vi "Send and Receive Example.vi"(0 "Input Data":T1 {"Command" format="%02x"; "Destination" format="%02x"; "Source" format="%02x"}, 1 "Read Timeout (ms)":u32=500, 5 "Expected Command":string=".*", 7 "Expected Data":string=".*", 11 "Error In":errorcluster) -> (4 "Raw Data Out":string, 6 "Coverted Data Out":T2 {"CRC" format="%04x"; "Length" format="%02x"; "Command" format="%02x"; "Destination" format="%02x"; "Source" format="%02x"}, 15 "Error Out":errorcluster)   [LabVIEW 2016]
doc: "This standalone VI sends a GEA2 message and returns the very next response."
uses:
  type defs/Data Out.ctl
  type defs/Data In.ctl
  library/GEA2_Toolkit.lvlib
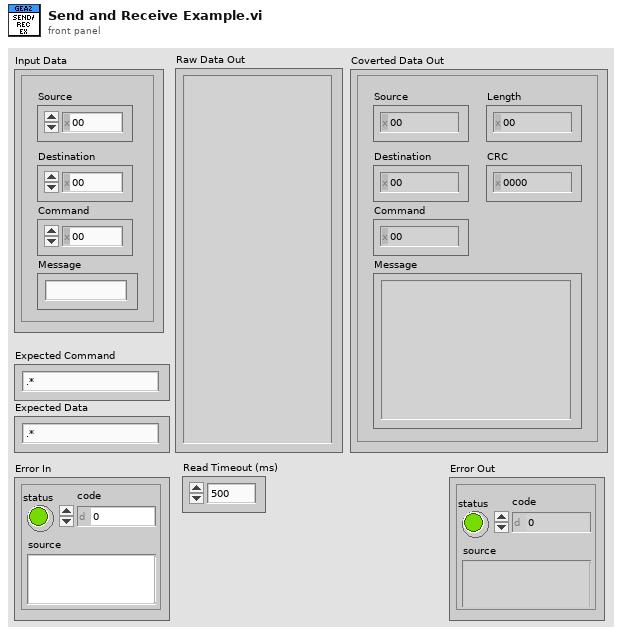
[diagram p1: front panel]
types:
  T1 = typedef "GEA2_Toolkit.lvlib/Data In.ctl" = cluster{"Source":u8, "Destination":u8, "Command":u8, "Message":string}
  T2 = typedef "GEA2_Toolkit.lvlib/Data Out.ctl" = cluster{"Source":u8, "Destination":u8, "Command":u8, "Length":u8, "CRC":u16, "Message":string}
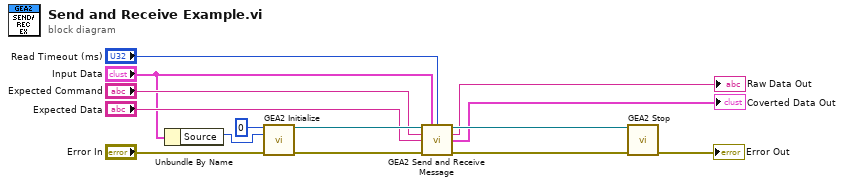
[diagram p0: block diagram]
diagram:
  n1 = Unbundle By Name("Input Data") -> ("Source"=w1:u8)
  n2 = call "GEA2 Initialize.vi"("Board Index"=0, "Source Address"=w1, "error in"="Error In") -> ("GEA2 Reference Out"=w14:refnum<k24>, "error out"=w11:errorcluster)  [unwired: 10 in, 1 out]
  n3 = call "GEA2 Send and Receive Message.vi"("GEA2 Reference In"=w14, "Input Data"="Input Data", "Read Timeout (ms)"="Read Timeout (ms)", "Expected Command"="Expected Command", "Expected Data"="Expected Data", "Error In"=w11) -> ("GEA2 Reference Out"=w13:refnum<k24>, "Raw Data Out"=→"Raw Data Out":string, "Converted Data Out"=→"Coverted Data Out":T2, "Error Out"=w12:errorcluster)  [unwired: 4 in, 2 out]
  n4 = call "GEA2 Stop.vi"("GEA2 Reference Out"=w13, "Error In"=w12) -> ("Error Out"=→"Error Out":errorcluster)  [unwired: 13 in]
